vi "MichaelTeleop.vi"(10 "Match Info":T1={"Autonomous Elapsed Seconds"=0.0, "TeleOp Elapsed Seconds"=0.0, "Disabled Elapsed Seconds"=0.0, "Visited Autonomous"=FALSE, "Visited TeleOp"=FALSE, "Visited Disabled"=FALSE, "Autonomous Settings"={"Autonomous Style"=enum."Independent", "VI Refnum"=refnum}}, 11 "Call Context":T2) -> ()   [LabVIEW 2017]
doc: "This VI is called for each TeleOp packet received from the DS where the robot is not disabled. It is often used to read from the joysticks and update I/O or to update setpoints for timed control loops. It should complete and return within 20 milliseconds or it may miss DS packets."
uses:
  <vilib>/Rock Robotics/WPI/DriverStation/WPI_DriverStationDerivedRobotMode.ctl
  <vilib>/Rock Robotics/WPI/DriverStation/WPI_DriverStationMatch Info.ctl
  IntakeAngleState.ctl
  Lift States.ctl
  Robot Global Data.vi
  Joystick Values.vi
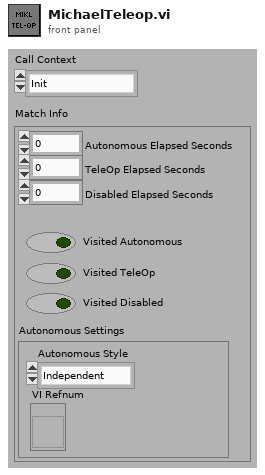
[diagram p1: front panel]
types:
  T1 = typedef "WPI_DriverStationMatch Info.ctl" = cluster{"Autonomous Elapsed Seconds":dbl, "TeleOp Elapsed Seconds":dbl, "Disabled Elapsed Seconds":dbl, "Visited Autonomous":bool, "Visited TeleOp":bool, "Visited Disabled":bool, "Autonomous Settings":cluster{"Autonomous Style":enum16{"Iterative", "Independent"}, "VI Refnum":refnum<vi>}}
  T2 = typedef "WPI_DriverStationDerivedRobotMode.ctl" = enum16{"Init", "Execute", "Stop"}
  T3 = typedef "Lift States.ctl" = enum16{"Manual", "Scale Low", "Scale Middle", "Scale High", "Rock Bottom", "Almost Down"}
  T4 = typedef "IntakeAngleState.ctl" = enum16{"Idle", "Manual", "Setpoint"}
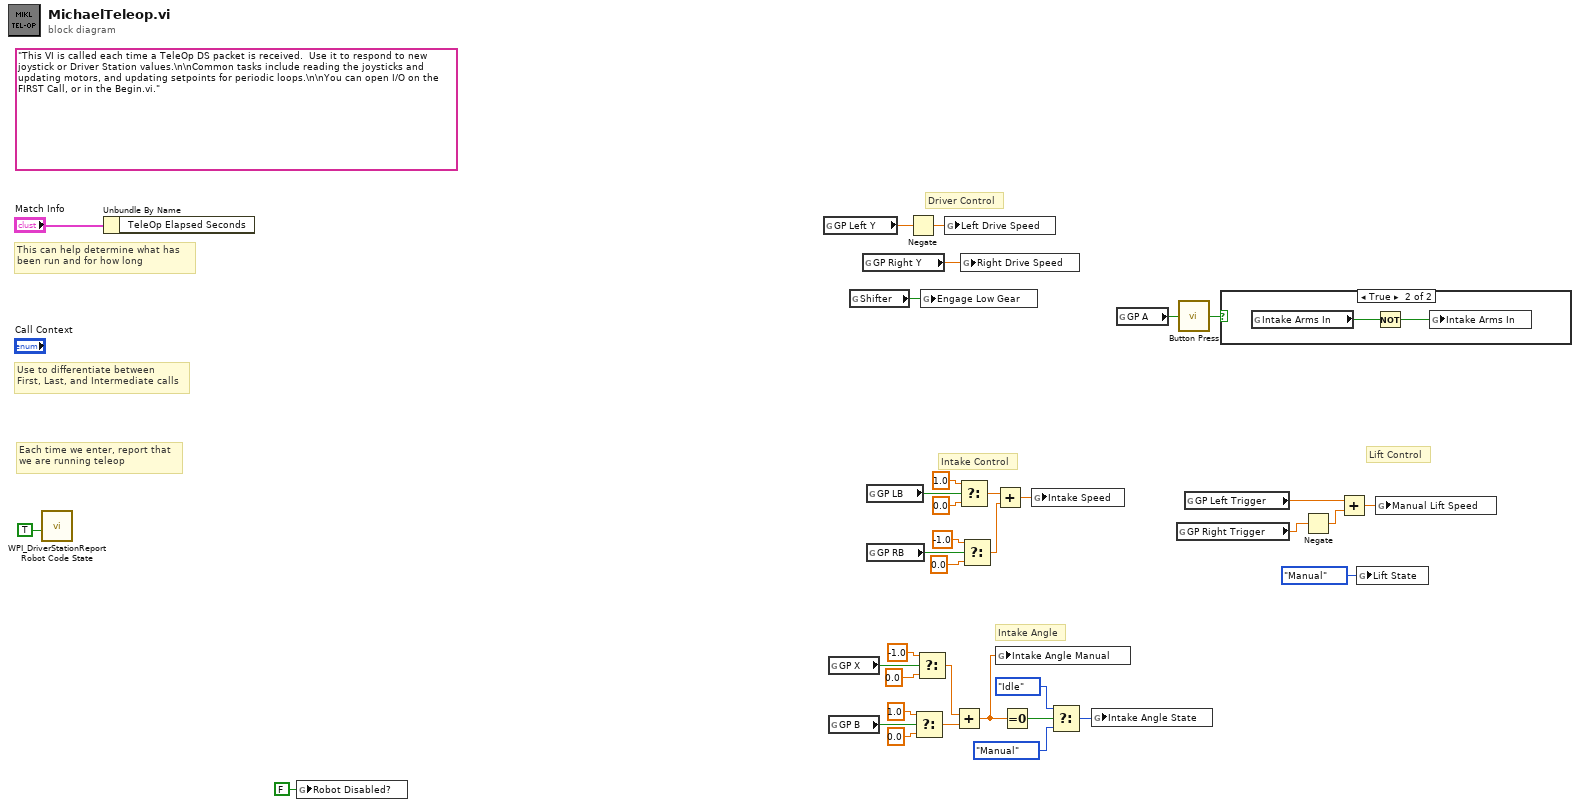
[diagram p0: block diagram]
diagram:
  (unwired) "This VI is called each time a TeleOp DS packet is received.  Use it to respond to new joystick or Driver Station values.\n\nCommon tasks include reading the joysticks and updating motors, and updating setpoints for periodic loops.\n\nYou can open I/O on the FIRST Call, or in the Begin.vi."
  # "Intake Angle"
  # "Lift Control"
  # "Driver Control"
  # "Intake Control"
  # "Each time we enter, report that\nwe are running teleop"
  # "Use to differentiate between\nFirst, Last, and Intermediate calls"
  # "This can help determine what has\nbeen run and for how long"
  n1 = call <vilib>:"WPI_DriverStationReport Robot Code State.vi"("TeleOp"=TRUE ("Autonomous")) -> ()  [unwired: 10 in, 1 out]
  n2 = Unbundle By Name("Match Info") -> ()  [unwired: 1 out]
  n3 = global write "Robot Global Data.vi" "Robot Disabled?"(FALSE ("AUTO Start Left")) -> ()
  n4 = global read "Joystick Values.vi" "GP Left Y"() -> (w30:dbl)
  n5 = global read "Joystick Values.vi" "GP X"() -> (w11:bool)
  n6 = global read "Joystick Values.vi" "GP B"() -> (w12:bool)
  n7 = global read "Joystick Values.vi" "Shifter"() -> (w28:bool)
  n8 = global read "Joystick Values.vi" "GP Right Y"() -> (w31:dbl)
  n9 = global read "Joystick Values.vi" "GP LB"() -> (w21:bool)
  n10 = global read "Joystick Values.vi" "GP RB"() -> (w18:bool)
  n11 = Negate(x=w30) -> (-x=w29:dbl)
  n12 = Select(t=1.0, s=w12, f=0.0) -> (s? t:f=w5:dbl)
  n13 = Select(t=-1.0, s=w11, f=0.0) -> (s? t:f=w6:dbl)
  n14 = global write "Robot Global Data.vi" "Engage Low Gear"(w28) -> ()
  n15 = global write "Robot Global Data.vi" "Left Drive Speed"(w29) -> ()
  n16 = Add(x=w6, y=w5) -> (x+y=w26:dbl)
  n17 = Select(t=1.0, s=w21, f=0.0) -> (s? t:f=w16:dbl)
  n18 = global write "Robot Global Data.vi" "Right Drive Speed"(w31) -> ()
  n19 = Select(t=-1.0, s=w18, f=0.0) -> (s? t:f=w15:dbl)
  n20 = Add(x=w16, y=w15) -> (x+y=w14:dbl)
  n21 = global write "Robot Global Data.vi" "Intake Angle Manual"(w26) -> ()
  n22 = Equal To 0?(x=w26) -> (x = 0?=w25:bool)
  n23 = global write "Robot Global Data.vi" "Intake Speed"(w14) -> ()
  n24 = Select(t=IntakeAngleState."Idle" ("Cube State"), s=w25, f=IntakeAngleState."Manual") -> (s? t:f=w23:T4)
  n25 = global write "Robot Global Data.vi" "Intake Angle State"(w23) -> ()
  n26 = global read "Joystick Values.vi" "GP A"() -> (w33:bool)
  n27 = global read "Joystick Values.vi" "GP Right Trigger"() -> (w3:dbl)
  n28 = call "Button Press.vi"("Current Button"=w33) -> ("Pressed?"=w32:bool)
  n29 = global read "Joystick Values.vi" "GP Left Trigger"() -> (w1:dbl)
  n30 = case shown="True" w32 {
    frame False {
    }
    frame True {
      n31 = global read "Robot Global Data.vi" "Intake Arms In"() -> (w38:bool)
      n32 = Not(x=w38) -> (.not. x?=w37:bool)
      n33 = global write "Robot Global Data.vi" "Intake Arms In"(w37) -> ()
    }
  }
  n34 = Negate(x=w3) -> (-x=w2:dbl)
  n35 = Add(x=w1, y=w2) -> (x+y=w13:dbl)
  n36 = global write "Robot Global Data.vi" "Lift State"(Lift_States."Manual" ("Lift State")) -> ()
  n37 = global write "Robot Global Data.vi" "Manual Lift Speed"(w13) -> ()
